vi "computecell.vi"(8 "i2":i32, 11 "i1":i32) -> (3 "Cell rect":cluster{dbl, dbl, dbl, dbl})   [LabVIEW 2023]
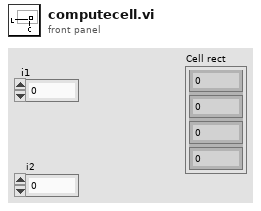
[diagram p1: front panel]
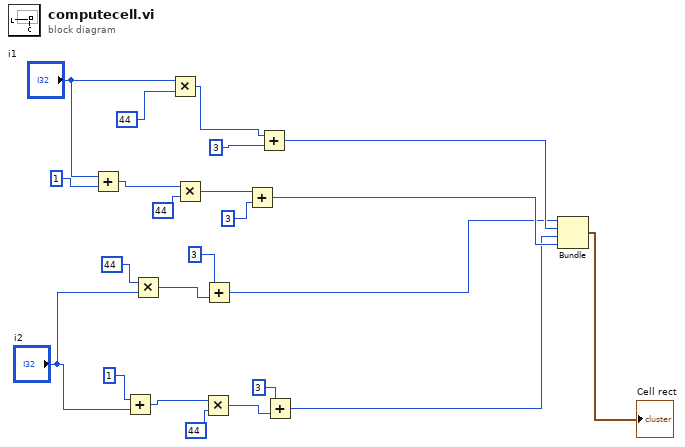
[diagram p0: block diagram]
diagram:
  n1 = Add(x="i1", y=1) -> (x+y=w17:i32)
  n2 = Add(x=1, y="i2") -> (x+y=w6:i32)
  n3 = Multiply(x=44, y="i2") -> (x*y=w10:i32)
  n4 = Multiply(x="i1", y=44) -> (x*y=w21:i32)
  n5 = Multiply(x=w17, y=44) -> (x*y=w14:i32)
  n6 = Multiply(x=w6, y=44) -> (x*y=w4:i32)
  n7 = Add(x=3, y=w10) -> (x+y=w8:i32)
  n8 = Add(x=w14, y=3) -> (x+y=w12:i32)
  n9 = Add(x=w21, y=3) -> (x+y=w13:i32)
  n10 = Add(x=3, y=w4) -> (x+y=w2:i32)
  n11 = Bundle(w8, w13, w2, w12) -> (→"Cell rect":cluster{i32, i32, i32, i32})  [unwired: 1 in]
